vi "P11Y2MRWORLDWIDE.vi"() -> ()   [LabVIEW 2020]
panel:
  out "GlobaalneArv":dbl
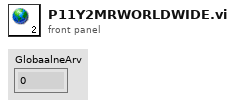
[diagram p1: front panel]
diagram:
